vi "Test logger.vi"(8 "error in":errorcluster, 10 "text":string) -> (0 "error out":errorcluster)   [LabVIEW 2014, in "UEGO Sim Engine.lvlib"]
uses:
  UEGO Sim Engine.lvlib
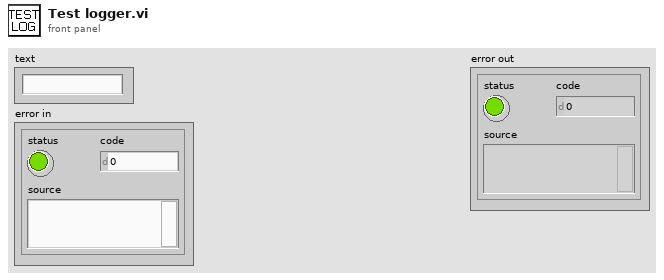
[diagram p1: front panel]
types:
  T1 = enum16{"open", "replace", "create", "open or create", "replace or create", "replace or create with confirmation"}
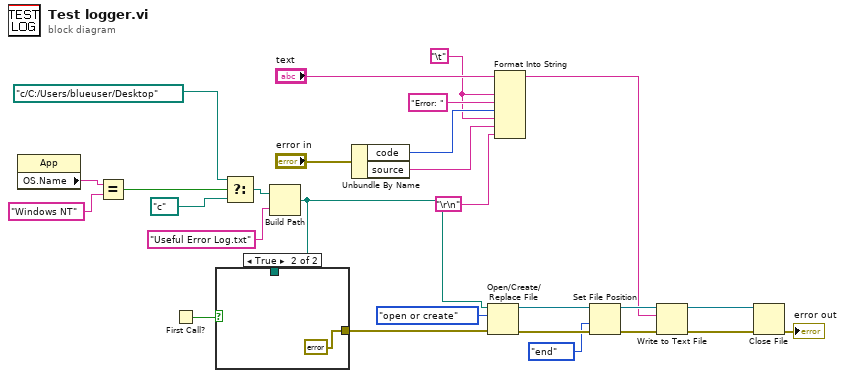
[diagram p0: block diagram]
diagram:
  w12 = "\t"
  n1 = property class="App"() -> ("OS.Name"=w7:string)  [unwired: 2 in, 2 out]
  n2 = Equal?(x=w7, y="Windows NT") -> (x = y?=w5:bool)
  n3 = First Call?() -> (First Call?: T/F=w19:bool)
  n4 = Select(t=path "c:/C:/Users/blueuser/Desktop", s=w5, f=path "c:/") -> (s? t:f=w3:path)
  n5 = Build Path(base path=w3, name or relative path="Useful Error Log.txt") -> (appended path=w1:path)
  n6 = case shown="True" w19 {
    tunnel: w1 -> [_ _]
    tunnel: [_ errorcluster {"status"=FALSE, "code"=0, "source"=""} ("error out")] -> w18
    frame False {
    }
    frame True {
    }
  }
  n7 = Unbundle By Name("error in") -> ("code"=w13:i32, "source"=w11:string)
  n8 = Open/Create/Replace File(file path (use dialog)=w1, error in=w18, operation (0:open)=T1."open or create") -> (refnum out=w26:refnum<file>, error out=w25:errorcluster)  [unwired: 3 in, 1 out]
  n9 = Format Into String(initial string="text", w12, "Error: ", w13, w12, w11, "\r\n") -> (resulting string=w9:string)  [unwired: 2 in, 1 out]
  n10 = Set File Position(refnum=w26, from (0:start)=enum16{"start", "end", "current"}."end", error in=w25) -> (refnum out=w22:refnum<file>, error out=w23:errorcluster)  [unwired: 1 in]
  n11 = Write to Text File(file (use dialog)=w22, text=w9, error in=w23) -> (refnum out=w20:refnum<file>, error out=w21:errorcluster)  [unwired: 1 in, 1 out]
  n12 = Close File(refnum=w20, error in=w21) -> (error out=→"error out":errorcluster)  [unwired: 1 out]
